vi "Config-Output-Sequence.vi"(8 "error in (no error)":errorcluster, 10 "output sequence":u16[](array[ring])=[0, 1, 2, 3, 6, 7] items=["SMU1", "SMU2", "SMU3", "SMU4", "SMU5", "SMU6", "VSU1", "VSU2", "PGU1", "PGU2"], 11 "VISA session":refnum<visa-resource-name>) -> (0 "error out":errorcluster, 3 "VISA resource name out":refnum<visa-resource-name>)   [LabVIEW 2016, in "Agilent 415X Series.lvlib"]
doc: "This VI configures the sequence of the units' output.\n\n* Currently there is a problem with the commands used by this VI. In order to set a sequence, this VI needs to be run once, and the user then need to select LOCAL using the push button on the front panel of the instrument. Then the second run of this VI will set the sequence."
uses:
  Agilent 415X Series.lvlib
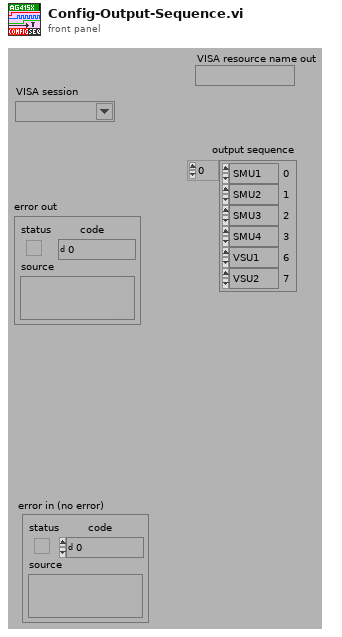
[diagram p1: front panel]
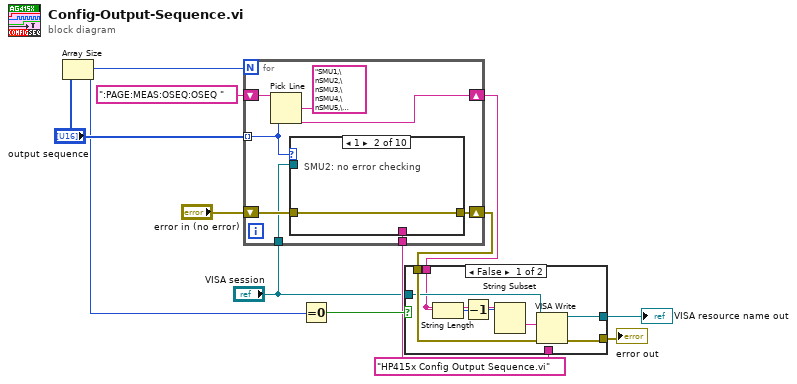
[diagram p0: block diagram]
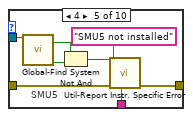
[diagram p6: hidden frame]
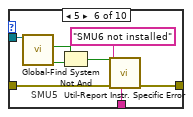
[diagram p7: hidden frame]
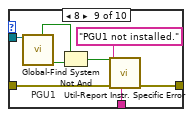
[diagram p10: hidden frame]
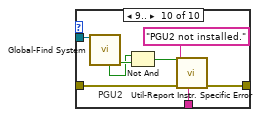
[diagram p11: hidden frame]
diagram:
  w4 = "HP415x Config Output Sequence.vi"
  n1 = Array Size(array="output sequence") -> (size(s)=w8:i32)
  n2 = for {
    N: w8 -> [_]
    tunnel: "output sequence" -> [w16] mode=indexing
    shift-right: [w14] -> w6
    shift-left: "error in (no error)" -> [w15]
    shift-right: [w17] -> w5
    shift-left: ":PAGE:MEAS:OSEQ:OSEQ " -> [w19]
    tunnel: "VISA session" -> [w13]
    tunnel: w4 -> [w12]
    n3 = Pick Line(string ("")=w19, multi-line string="SMU1,\nSMU2,\nSMU3,\nSMU4,\nSMU5,\nSMU6,\nVSU1,\nVSU2,\nPGU1,\nPGU2,", line index=w16) -> (output string=w17:string)
    n4 = case shown="1" w16 {
      tunnel: w15 -> [w20 w21 w22 w23 w27 w36 w40 w41 w46 w54]
      tunnel: [w20 w21 w22 w23 w26 w35 w40 w41 w45 w53] -> w14
      tunnel: w13 -> [_ _ _ _ w31 w39 _ _ w49 w57]
      tunnel: w12 -> [_ _ _ _ w25 w34 _ _ w44 w52]
      frame ..0 {
        # "SMU1: no error checking"
      }
      frame 1 {
        # "SMU2: no error checking"
      }
      frame 2 {
        # "SMU3: no error checking"
      }
      frame 3 {
        # "SMU4: no error checking"
      }
      frame 4 {
        # "SMU5"
        n5 = call "Global-Find System.vi"("VISA session"=w31) -> ("found"=w29:bool, "SMU5 present"=w30:bool)  [unwired: 3 in, 6 out]
        n6 = Not And(1:w29, 2:w30) -> (0:w28:bool)
        n7 = call "Util-Report Instr. Specific Error.vi"("source"=w25, "error in (no error)"=w27, "error message"="SMU5 not installed", "new error"=w28) -> ("error out"=w26:errorcluster)  [unwired: 6 in, 1 out]
      }
      frame 5 {
        # "SMU5"
        n8 = call "Global-Find System.vi"("VISA session"=w39) -> ("found"=w38:bool, "SMU6 present"=w32:bool)  [unwired: 3 in, 6 out]
        n9 = Not And(1:w38, 2:w32) -> (0:w37:bool)
        n10 = call "Util-Report Instr. Specific Error.vi"("source"=w34, "error in (no error)"=w36, "error message"="SMU6 not installed", "new error"=w37) -> ("error out"=w35:errorcluster)  [unwired: 6 in, 1 out]
      }
      frame 6 {
        # "VSU1: no error checking"
      }
      frame 7 {
        # "VSU2: no error checking"
      }
      frame 8 {
        # "PGU1"
        n11 = call "Global-Find System.vi"("VISA session"=w49) -> ("found"=w48:bool, "PGU1 present"=w42:bool)  [unwired: 3 in, 6 out]
        n12 = Not And(1:w48, 2:w42) -> (0:w47:bool)
        n13 = call "Util-Report Instr. Specific Error.vi"("source"=w44, "error in (no error)"=w46, "error message"="PGU1 not installed.", "new error"=w47) -> ("error out"=w45:errorcluster)  [unwired: 6 in, 1 out]
      }
      frame 9.. {
        # "PGU2"
        n14 = call "Global-Find System.vi"("VISA session"=w57) -> ("found"=w56:bool, "PGU2 present"=w50:bool)  [unwired: 3 in, 6 out]
        n15 = Not And(1:w56, 2:w50) -> (0:w55:bool)
        n16 = call "Util-Report Instr. Specific Error.vi"("source"=w52, "error in (no error)"=w54, "error message"="PGU2 not installed.", "new error"=w55) -> ("error out"=w53:errorcluster)  [unwired: 6 in, 1 out]
      }
    }
  }
  n17 = Equal To 0?(x=w8) -> (x = 0?=w7:bool)
  n18 = case shown="False" w7 {
    tunnel: w6 -> [w64 w67]
    tunnel: w5 -> [w60 _]
    tunnel: w4 -> [_ _]
    tunnel: "VISA session" -> [w63 w66]
    tunnel: [w65 w67] -> w2
    tunnel: [w58 w66] -> w1
    frame False {
      n19 = String Length(string=w60) -> (length=w61:i32)
      n20 = Decrement(x=w61) -> (x-1=w59:i32)
      n21 = String Subset(string=w60, length (rest)=w59) -> (substring=w62:string)  [unwired: 1 in]
      n22 = VISA Write(VISA resource name=w63, write buffer=w62, error in (no error)=w64) -> (VISA resource name out=w58:refnum<visa-resource-name>, error out=w65:errorcluster)  [unwired: 1 out]
    }
    frame True {
    }
  }
  "error out" <- w2
  "VISA resource name out" <- w1
